vi "Close.vi"(0 "disk streaming in":refnum<class "Disk Streaming.lvclass">, 5 "error in (no error)":errorcluster) -> (19 "error out":errorcluster)   [LabVIEW 2021, in "Disk Streaming.lvclass"]
doc: "Closes the disk streaming instance created by the <B>Open.vi</B>, and the TDMS file used by the instance.\n\nInputs:\n\n<B>disk streaming in</B>: Disk streaming instance input."
uses:
  Disk Streaming.lvclass
  Disk Streaming.lvclass/Disk Streaming.ctl
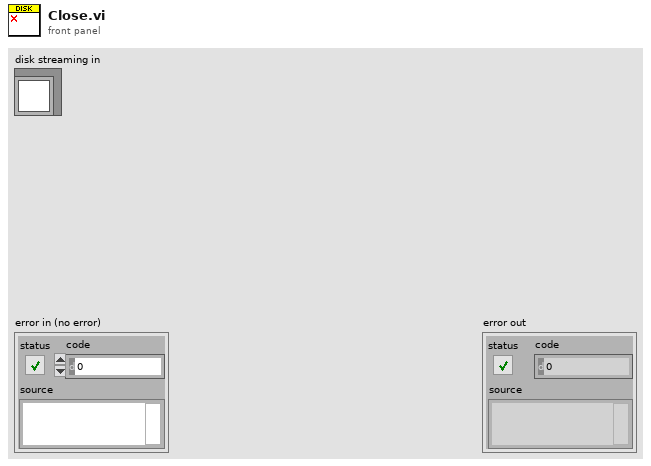
[diagram p1: front panel]
types:
  T1 = typedef "Disk Streaming.lvclass/Data.ctl" = cluster{"tdms file":refnum<k34>, "group name":string, "channel name":string, "max operations":u32, "timeout (s)":dbl, "data type size (bytes)":u64, "writing":bool, "I/O mode":T2, "# of blocks":u32, "block size divisor (bytes)":u32, "file position (elements)":u64, "file size (elements)":i64, "file size (samples)":i64, "block size (elements)":u64, "block size (samples)":u64, "quantum size (elements)":u64, "quantum size (samples)":u64, "samples remaining":i64, "elements transferred":u64, "finished":bool, "preview size":i32, "preview quantum size (elements)":u64, "preview quantum size (samples)":u64, "DMA buffer size (elements)":u32, "pending block sizes (bytes)":u64[]}
  T2 = typedef "Disk Streaming.lvclass/IO mode.ctl" = enum16{"Synchronous", "Asynchronous", "Data Reference"}
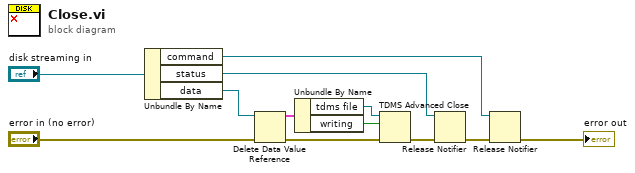
[diagram p0: block diagram]
diagram:
  n1 = Unbundle By Name("disk streaming in") -> ("command"=w3:refnum<notifier>, "status"=w5:refnum<notifier>, "data"=w10:refnum<data-value>)
  n2 = Delete Data Value Reference(data value reference=w10, error in="error in (no error)") -> (data value=w9:T1, error out=w8:errorcluster)
  n3 = Unbundle By Name(w9) -> ("tdms file"=w7:refnum<k34>, "writing"=w1:bool)
  n4 = TDMS Advanced Close(8:w8, 10:w1, 11:w7) -> (0:w6:errorcluster)  [unwired: 1 in, 1 out]
  n5 = Release Notifier(notifier=w5, error in (no error)=w6) -> (error out=w4:errorcluster)  [unwired: 1 in, 2 out]
  n6 = Release Notifier(notifier=w3, error in (no error)=w4) -> (error out=→"error out":errorcluster)  [unwired: 1 in, 2 out]
